vi "Get Log File Auto Open.vi"(8 "error in":errorcluster, 11 "log file in":T1 format="%.0x") -> (0 "error out":errorcluster, 2 "auto open":bool, 3 "log file out":T1 format="%.0x")   [LabVIEW 2027, in "Embedded Data Logger Scripting.lvlib"]
uses:
  Embedded Data Logger Scripting.lvlib
  <vilib>/NI VeriStand/Custom Device API/Custom Device Item Ref.ctl
  <vilib>/NI VeriStand/Custom Device API/Get Item Property (Boolean).vi
  <vilib>/NI VeriStand/Custom Device API/Custom Device API.lvlib
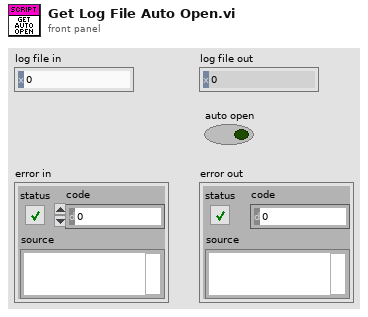
[diagram p1: front panel]
types:
  T1 = typedef "Custom Device API.lvlib/Custom Device Item Ref.ctl" = u64
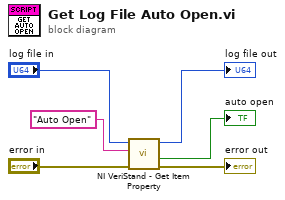
[diagram p0: block diagram]
diagram:
  n1 = call-poly <vilib>:"NI VeriStand - Get Item Property.vi"("error in (no error)"="error in", "Property Name"="Auto Open", "Item Ref in"="log file in") -> ("error out"=→"error out":errorcluster, "Value"=→"auto open":bool, "Item Ref out"=→"log file out":T1)  [unwired: 1 in, 5 out]
